vi "get internal stream size.vi"(8 "error im":errorcluster, 11 "socket":u64) -> (0 "error out":errorcluster, 3 "size":u64)   [LabVIEW 2016, in "async tls dl.lvlib"]
uses:
  async tls dl.lvlib
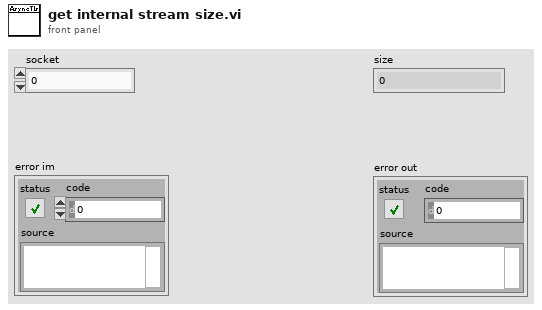
[diagram p1: front panel]
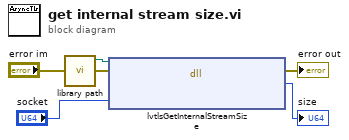
[diagram p0: block diagram]
diagram:
  n1 = call "library path.vi"() -> ("path"=w1:path)  [unwired: 11 in]
  n2 = dll-call lib="C:/Users/IEUser/Desktop/libasynclvtls/lvasynctls.dll" fn="lvtlsGetInternalStreamSize"(path in=w1, error in="error im", "socket"="socket") -> (error out=→"error out":errorcluster, "size"=→"size":u64)  [unwired: 2 in, 1 out]
